vi "localeSystemDecimalReplace (SubVI).vi"(11 "String":string) -> (3 "result string":string)   [LabVIEW 2017, in "LV_Unicorn.lvlib"]
uses:
  LV_Unicorn.lvlib
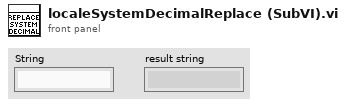
[diagram p1: front panel]
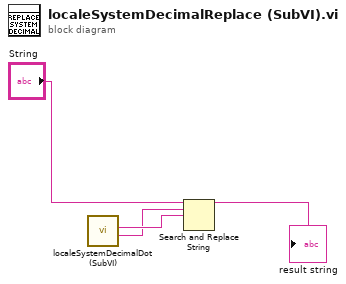
[diagram p0: block diagram]
diagram:
  n1 = call "localeSystemDecimalDot (SubVI).vi"() -> ("InvlocaleSystemDecimal"=w2:string, "localeSystemDecimal"=w3:string)  [unwired: 9 in, 1 out]
  n2 = Search and Replace String(input string="String", search string=w2, replace string=w3) -> (result string=→"result string":string)  [unwired: 5 in, 3 out]
